vi "Append (single).vi"(6 "Reset":bool, 8 "error in (no error)":errorcluster, 10 "XY-data (B)":cluster{"X-array":dbl[], "Y-array":dbl[]}, 11 "XY-data (A)":cluster{"X-array":dbl[], "Y-array":dbl[]}) -> (0 "error out":errorcluster, 3 "XY-data out":cluster{"X-array":dbl[], "Y-array":dbl[]} {"Y-array" format="%.2p"; "X-array" format="%.2p"})   [LabVIEW 2019, in "xy_utilities.lvlib"]
doc: "Append <B>XY-Data B</B> to the end of <B>XY-Data A</B> (similar to Append Waveforms.vi).\n\nWire data to the data input to determine the polymorphic instance to use or manually select the instance."
uses:
  xy_utilities.lvlib
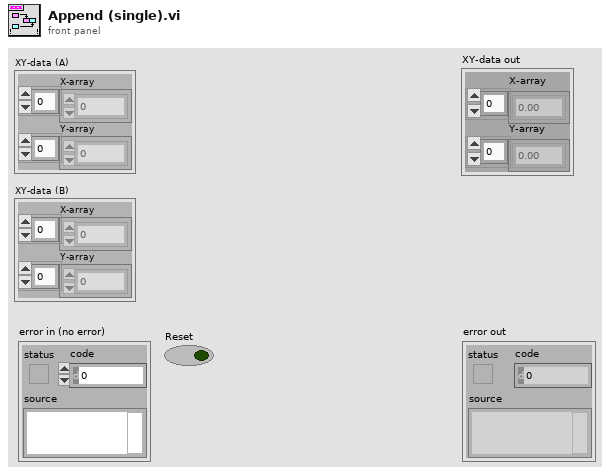
[diagram p1: front panel]
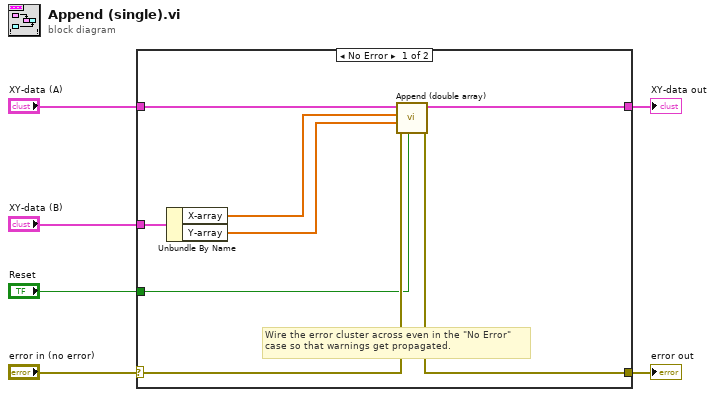
[diagram p0: block diagram]
diagram:
  n1 = case shown="No Error" "error in (no error)" {
    selector: "error in (no error)" -> [w10 w16]
    tunnel: [w9 w16] -> w5
    tunnel: "XY-data (A)" -> [w13 w15]
    tunnel: [w12 w15] -> w3
    tunnel: "XY-data (B)" -> [w14 _]
    tunnel: "Reset" -> [w7 _]
    frame No Error {
      # "Wire the error cluster across even in the \"No Error\"\ncase so that warnings get propagated."
      n2 = Unbundle By Name(w14) -> ("X-array"=w11:dbl[], "Y-array"=w8:dbl[])
      n3 = call "Append (double array).vi"("Reset"=w7, "error in (no error)"=w10, "Y-array"=w8, "X-array"=w11, "XY-data (A)"=w13) -> ("error out"=w9:errorcluster, "XY-data out"=w12:cluster{"X-array":dbl[], "Y-array":dbl[]})  [unwired: 5 in]
    }
    frame Error {
    }
  }
  "error out" <- w5
  "XY-data out" <- w3
